vi "ReadActiveDTCs.vi"(8 "error in (no error)":errorcluster, 9 "timeout ms (1000)":i32=1000, 10 "Options (KWP/UDS Only)":T1, 11 "Connection Info":T3) -> (0 "error out":errorcluster, 2 "Active DTCs":T2[](array[typedef]), 3 "Connection Info":T3)   [LabVIEW 2015, in "Diagnostics Host Automation API.lvlib"]
uses:
  Diagnostics Host Automation API.lvlib
  <userlib>/STM/TCP/stm_TCP Connection Info.ctl
  <userlib>/STM/_SubVIs/stm_MetaDataElement.ctl
  Shared/DTC and Timestamp Cluster.ctl
  Shared/RequestResponse Data Cluster.ctl
  <userlib>/STM/TCP/stm_TCP Write Options.ctl
  <userlib>/STM/TCP/STM Write Message (TCP).vi
  <userlib>/STM/TCP/STM Read Message (TCP).vi
  Shared/Diagnostics Addon Shared.lvlib
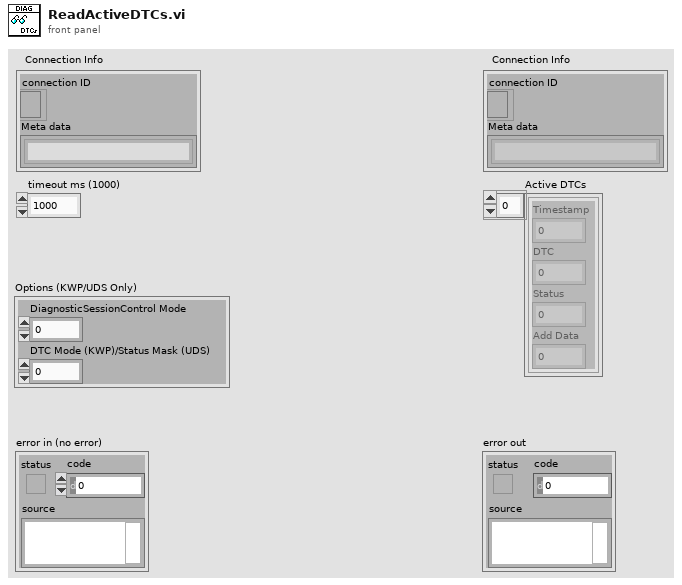
[diagram p1: front panel]
types:
  T1 = cluster{"DiagnosticSessionControl Mode":u8, "DTC Mode (KWP)/Status Mask (UDS)":u8}
  T2 = typedef "Diagnostics Addon Shared.lvlib/DTC and Timestamp Cluster.ctl" = cluster{"Timestamp":dbl, "DTC":dbl, "Status":dbl, "Add Data":dbl}
  T3 = typedef "stm_TCP Connection Info.ctl" = cluster{"connection ID":refnum<k5>, "Meta data":T4[]}
  T4 = typedef "stm_MetaDataElement.ctl" = string
  T5 = typedef "stm_TCP Write Options.ctl" = cluster{"Ignore Timeout Error":bool, "timeout ms (1000)":i32}
  T6 = typedef "Diagnostics Addon Shared.lvlib/RequestResponse Data Cluster.ctl" = cluster{"Timeout":i32, "data":string}
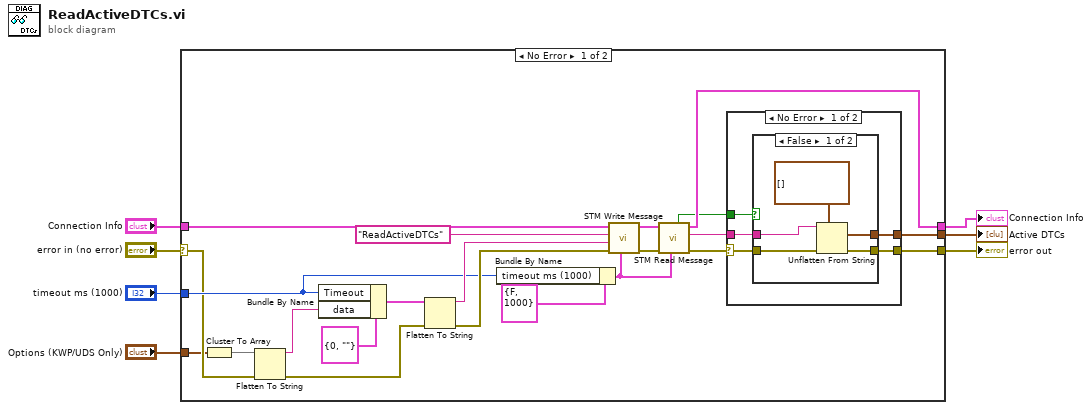
[diagram p0: block diagram]
diagram:
  n1 = case shown="No Error" "error in (no error)" {
    selector: "error in (no error)" -> [w12 w43]
    tunnel: "Connection Info" -> [w29 w42]
    tunnel: [w26 w42] -> w6
    tunnel: [w15 w43] -> w5
    tunnel: "timeout ms (1000)" -> [w19 _]
    tunnel: [w13 _] -> w2
    tunnel: "Options (KWP/UDS Only)" -> [w10 _]
    frame No Error {
      n2 = Cluster To Array(cluster=w10) -> (array=w8:u8[])
      n3 = Flatten To String(anything=w8, error in (no error)=w12) -> (data string=w9:string, error out=w11:errorcluster)  [unwired: 2 in, 1 out]
      n4 = Bundle By Name(cluster=T6 {"Timeout"=0, "data"=""}, "Timeout"=w19, "data"=w9) -> (w23:T6)
      n5 = Flatten To String(anything=w23, error in (no error)=w11) -> (data string=w21:string, error out=w22:errorcluster)  [unwired: 2 in, 1 out]
      n6 = Bundle By Name(cluster=T5 {"Ignore Timeout Error"=FALSE, "timeout ms (1000)"=1000} ("Options"), "timeout ms (1000)"=w19) -> (w18:T5)
      n7 = call-poly <userlib>:"STM Write Message.vi"("Options"=w18, "error in (no error)"=w22, "Data"=w21, "Name"="ReadActiveDTCs", "Connection Info"=w29) -> ("error out"=w25:errorcluster, "Connection Info Out"=w27:T3)  [unwired: 5 in]
      n8 = call-poly <userlib>:"STM Read Message.vi"("Options"=w18, "error in"=w25, "Connection Info"=w27) -> ("error out"=w17:errorcluster, "data string"=w14:string, "Connection Info Out"=w26:T3, "Timed Out?"=w16:bool)  [unwired: 3 in, 2 out]
      n9 = case shown="No Error" w17 {
        selector: w17 -> [w32 w41]
        tunnel: w16 -> [w34 _]
        tunnel: [w33 w41] -> w15
        tunnel: w14 -> [w31 _]
        tunnel: [w30 _] -> w13
        frame No Error {
          n10 = case shown="False" w34 {
            tunnel: [w38 w40] -> w33
            tunnel: w32 -> [w39 w40]
            tunnel: w31 -> [w36 _]
            tunnel: [w35 _] -> w30
            frame False {
              n11 = Unflatten From String(type=T2[] [] ("Active DTCs"), binary string=w36, error in (no error)=w39) -> (value=w35:T2[], error out=w38:errorcluster)  [unwired: 2 in, 1 out]
            }
            frame True {
            }
          }
        }
        frame Error {
        }
      }
    }
    frame Error {
    }
  }
  "Connection Info" <- w6
  "error out" <- w5
  "Active DTCs" <- w2
